vi "comm_test.vi"() -> ()   [LabVIEW 2010, in "LightSourceAN191011Chameleon.lvclass"]
uses:
  LightSourceAN191011Chameleon.lvclass
  <vilib>/Instr/_visa.llb/VISA Configure Serial Port (Instr).vi
panel:
  out "error out":errorcluster
  out "read buffer":string
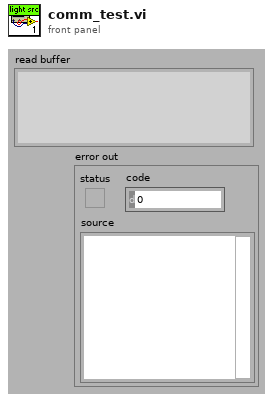
[diagram p1: front panel]
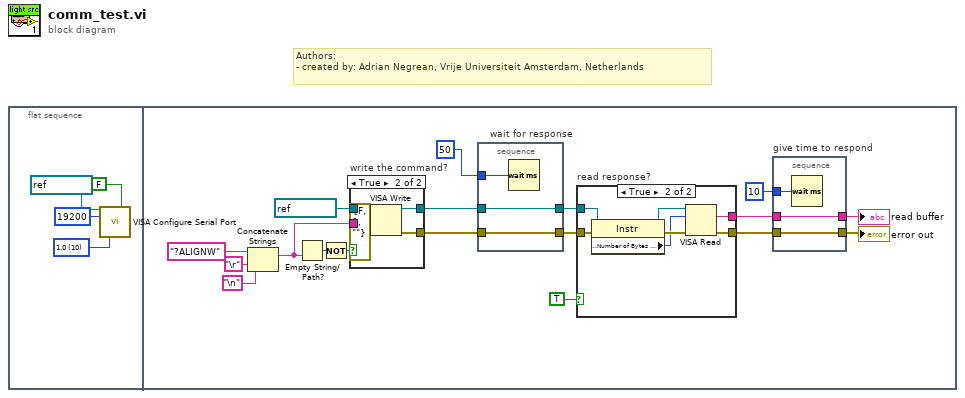
[diagram p0: block diagram]
diagram:
  # "Authors: \n- created by: Adrian Negrean, Vrije Universiteit Amsterdam, Netherlands"
  n1 = flat-sequence {
    frame #0 {
      w1 = u16 10 items=["1.0"=10, "1.5"=15, "2.0"=20] ("stop bits (10: 1 bit)")
      n2 = call-poly "VISA Configure Serial Port"("VISA resource name"=refnum<visa-resource-name> "COM4", "Enable Termination\nChar (T)"=FALSE ("Enable Termination\nChar (T)"), "baud rate (9600)"=u32 19200, "stop bits (10: 1 bit)"=w1) -> ()  [unwired: 10 in, 2 out]
    }
    frame #1 {
      n3 = Concatenate Strings("?ALIGNW" ("string"), "\r", "\n") -> (w19:string)
      n4 = Empty String/Path?(string/path=w19) -> (empty?=w20:bool)
      n5 = Not(x=w20) -> (.not. x?=w11:bool)
      n6 = case "write the command?" shown="True" w11 {
        tunnel: [_ w42] -> w17
        tunnel: [w37 w41] -> w18
        tunnel: refnum<visa-resource-name> "COM4" ("comm port") -> [w37 w40]
        tunnel: w19 -> [_ w39]
        frame False {
        }
        frame True {
          n7 = VISA Write(VISA resource name=w40, write buffer=w39, error in (no error)=errorcluster {"status"=FALSE, "code"=0, "source"=""}) -> (VISA resource name out=w41:refnum<visa-resource-name>, error out=w42:errorcluster)  [unwired: 1 out]
        }
      }
      n8 = stacked-sequence "wait for response" {
        tunnel: w17 -> [w36]
        tunnel: [w36] -> w12
        tunnel: w18 -> [w35]
        tunnel: [w35] -> w13
        tunnel: u32 50 ("milliseconds to wait") -> [w34]
        frame #0 {
          n9 = Wait (ms)(milliseconds to wait=w34) -> ()  [unwired: 1 out]
        }
      }
      n10 = case "read response?" shown="True" TRUE {
        tunnel: w12 -> [w26 w30]
        tunnel: [w26 w33] -> w16
        tunnel: w13 -> [_ w32]
        tunnel: [_ w27] -> w15
        frame False {
        }
        frame True {
          n11 = property class="Instr"(reference=w32, error in=w30) -> (reference out=w31:refnum<visa-resource-name>, error out=w29:errorcluster, "Serial Settings:Number of Bytes at Serial Port"=w28:u32)
          n12 = VISA Read(VISA resource name=w31, byte count=w28, error in (no error)=w29) -> (read buffer=w27:string, error out=w33:errorcluster)  [unwired: 2 out]
        }
      }
      n13 = stacked-sequence "give time to respond" {
        tunnel: w16 -> [w25]
        tunnel: [w25] -> w5
        tunnel: w15 -> [w24]
        tunnel: [w24] -> w6
        tunnel: u32 10 ("delay before read (ms)") -> [w23]
        frame #0 {
          n14 = Wait (ms)(milliseconds to wait=w23) -> ()  [unwired: 1 out]
        }
      }
      "read buffer" <- w6
      "error out" <- w5
    }
  }
